vi "Celsius_to_Farhenheit.vi"() -> ()   [LabVIEW 2015]
panel:
  out "Farhenheit":i32
  in  "Celsius":i32
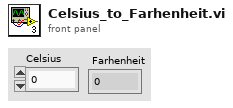
[diagram p1: front panel]
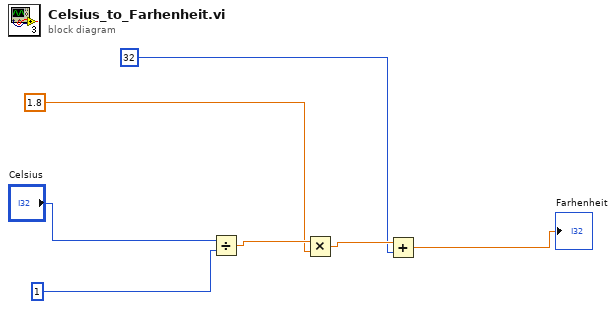
[diagram p0: block diagram]
diagram:
  n1 = Divide(x="Celsius", y=1) -> (x/y=w5:dbl)
  n2 = Multiply(x=w5, y=1.8) -> (x*y=w3:dbl)
  n3 = Add(x=w3, y=32) -> (x+y=→"Farhenheit":dbl)
